vi "configs.vi"() -> ()   [LabVIEW 2022 SP3]
uses:
  <vilib>/Utility/config.llb/NI_LVConfig.lvlib
panel:
  in  "Config File Path":path
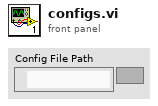
[diagram p1: front panel]
types:
  T1 = cluster{"Plot 1":cluster{"Name":string, "Sensors":i32[]}, "Plot 2":cluster{"Name":string, "Sensors":i32[]}, "Plot 3":cluster{"Name":string, "Sensors":i32[]}, "Plot 4":cluster{"Name":string, "Sensors":i32[]}}
  T2 = typedef "NI_LVConfig.lvlib/Config Data RefNum.ctl" = refnum<k1>
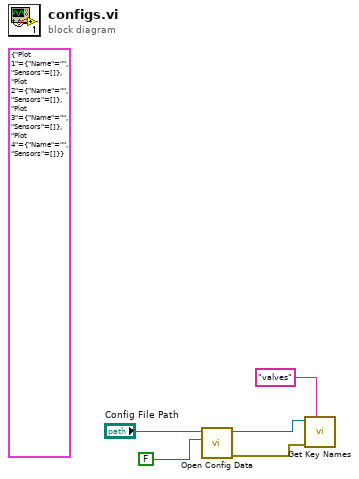
[diagram p0: block diagram]
diagram:
  (unwired) T1 {"Plot 1"={"Name"="", "Sensors"=[]}, "Plot 2"={"Name"="", "Sensors"=[]}, "Plot 3"={"Name"="", "Sensors"=[]}, "Plot 4"={"Name"="", "Sensors"=[]}}
  n1 = call <vilib>:"Open Config Data.vi"("create file if necessary (T)"=FALSE, "configuration file path"="Config File Path") -> ("error out"=w3:errorcluster, "refnum"=w2:T2)  [unwired: 7 in, 1 out]
  n2 = call <vilib>:"Get Key Names.vi"("section"="valves", "error in (no error)"=w3, "refnum"=w2) -> ()  [unwired: 5 in, 4 out]
